vi "PWM舵机驱动实验--基于底层驱动.vi"() -> ()   [LabVIEW 2011]
uses:
  <vilib>/STM32_DriverVI_Interface_F4/Timer/TIM4_Group_Pins_F4.ctl
  <vilib>/STM32_DriverVI_Interface_F4/Timer/TIM4_Channels_Pin_Map_F4.ctl
  <vilib>/STM32_DriverVI_Interface_F4/GPIO/GPIO_Group_Mode_Interface_F4.ctl
  <vilib>/STM32_DriverVI_Interface_F4/Timer/PWM Mode_F4.ctl
  <vilib>/STM32_DriverVI_Interface_F4/Timer/TIM4_PWM_Channel_F4.ctl
  <vilib>/STM32_DriverVI_Interface_F4/Timer/Reload Mode_F4.ctl
  <vilib>/STM32_DriverVI_Interface_F4/Timer/TIM4 Init_F4.vi
  <vilib>/STM32_DriverVI_Interface_F4/Timer/TIM4 Channel Pin Map_F4.vi
  <vilib>/STM32_DriverVI_Interface_F4/Timer/TIM4 PWM Mode Set_F4.vi
  <vilib>/STM32_DriverVI_Interface_F4/Timer/TIM4 PWM Permit_UnPermit_F4.vi
  <vilib>/STM32_DriverVI_Interface_F4/Timer/TIM4 Int Enable_Disable_F4.vi
  <vilib>/STM32_DriverVI_Interface_F4/Timer/TIM4_PWM_Update_Duty_F4.vi
panel:
  in  "仪表":u8(knob) scale=0.0..180.0
  out "数值":i32
  in  "停止":bool
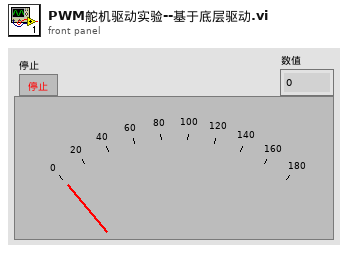
[diagram p1: front panel]
types:
  T1 = typedef "中断使能禁止.ctl" = enum8{"Disable", "Enable"}
  T2 = typedef "允许或禁止PWM输出_F4.ctl" = enum8{"禁止", "允许"}
  T3 = typedef "TIM4_PWM_Channel_F4.ctl" = enum8{"TIM4_Channel_1", "TIM4_Channel_2", "TIM4_Channel_3", "TIM4_Channel_4"}
  T4 = typedef "PWM Mode_F4.ctl" = enum16{"First Low Then High", "First High Then Low", "Output Match Mode"}
  T5 = typedef "GPIO_Group_Mode_Interface_F4.ctl" = enum8{"Floating Input", "Pull-up Input", "Pull-down Input", "-----------------------", "Push-pull Output", "Open-drain Output"}[]
  T6 = typedef "TIM4_Group_Pins_F4.ctl" = T7[]
  T7 = typedef "TIM4_Channels_Pin_Map_F4.ctl" = enum8{"TIM4_Channel_1-->PB6", "TIM4_Channel_1-->PD12", "TIM4_Channel_2-->PB7", "TIM4_Channel_2-->PD13", "TIM4_Channel_3-->PB8", "TIM4_Channel_3-->PD14", "TIM4_Channel_4-->PB9", "TIM4_Channel_4-->PD15", "TIM4_ETR-->PE0"}
  T8 = typedef "TIMX计数时钟频率_F4.ctl" = u16
  T9 = typedef "Reload Mode_F4.ctl" = enum8{"写入时立刻重载", "发生更新中断时重载"}
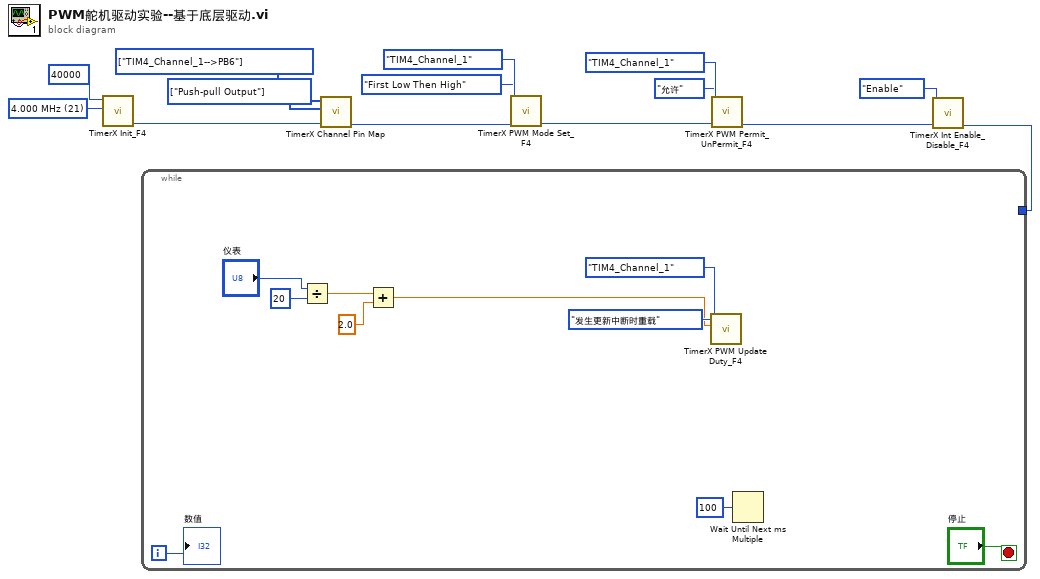
[diagram p0: block diagram]
diagram:
  w10 = T5 [enum."Push-pull Output"] items=["Floating Input", "Pull-up Input", "Pull-down Input", "-----------------------", "Push-pull Output", "Open-drain Output"] ("GPIO Mode Set")
  w11 = T6 [enum."TIM4_Channel_1-->PB6"] items=["TIM4_Channel_1-->PB6", "TIM4_Channel_1-->PD12", "TIM4_Channel_2-->PB7", "TIM4_Channel_2-->PD13", "TIM4_Channel_3-->PB8", "TIM4_Channel_3-->PD14", "TIM4_Channel_4-->PB9", "TIM4_Channel_4-->PD15", "TIM4_ETR-->PE0"] ("TIM4 Group Channel Pins")
  w13 = T8 21 items=["84.00 MHz"=1, "42.00 MHz"=2, "28.00 MHz"=3, "21.00 MHz"=4, "12.000 MHz"=7, "7.000 MHz"=12, "4.000 MHz"=21, "1.000 MHz"=84, "-------------"=0, "500.0 KHz"=168, "250.0 KHz"=336, "100.0 KHz"=840, "50.00 KHz"=1680, "10.00 KHz"=8400] ("时钟预分频数")
  n1 = call-poly <vilib>:"TimerX Init_F4.vi"("时钟预分频数"=w13, "自动重装值"=u16 40000) -> ("err_out"=w12:u8)  [unwired: 9 in]
  n2 = call-poly <vilib>:"TimerX Channel Pin Map.vi"("err_in"=w12, "GPIO Mode Set"=w10, "TIM4 Group Channel Pins"=w11) -> ("err_out"=w9:u8)  [unwired: 8 in]
  n3 = call-poly <vilib>:"TimerX PWM Mode Set_F4.vi"("err_in"=w9, "PWM Mode"=PWM_Mode_F4."First Low Then High", "TIM4_PWM_Channel"=TIM4_PWM_Channel_F4."TIM4_Channel_1") -> ("err_out"=w8:u8)  [unwired: 8 in]
  n4 = call-poly <vilib>:"TimerX PWM Permit_UnPermit_F4.vi"("err_in"=w8, "允许或禁止PWM输出"=允许或禁止PWM输出_F4."允许", "TIM4_PWM_Channel"=TIM4_PWM_Channel_F4."TIM4_Channel_1") -> ("err_out"=w3:u8)  [unwired: 8 in]
  n5 = call-poly <vilib>:"TimerX Int Enable_Disable_F4.vi"("err_in"=w3, "中断使能/关闭"=中断使能禁止."Enable") -> ("err_out"=w1:u8)  [unwired: 9 in]
  n6 = while {
    tunnel: w1 -> [_]
    i -> [w20]
    stop <- "停止" stop-if-true
    n7 = Divide(x="仪表", y=20) -> (x/y=w17:dbl)
    n8 = Add(x=w17, y=2.0) -> (x+y=w15:dbl)
    n9 = call-poly <vilib>:"TimerX PWM Update Duty_F4.vi"("占空比更新重载方式"=Reload_Mode_F4."发生更新中断时重载", "TIM4 PWM Duty（%）"=w15, "TIM4_PWM_Channel"=TIM4_PWM_Channel_F4."TIM4_Channel_1") -> ()  [unwired: 8 in, 1 out]
    n10 = Wait Until Next ms Multiple(millisecond multiple=u32 100 ("毫秒倍数")) -> ()  [unwired: 1 out]
    "数值" <- w20
  }
